vi "get current vi lib.vi"(8 "Stored Path":path) -> (0 "Current VI Lib Path":path)   [LabVIEW 2014, in "PL Framework Configuration Tool.lvlib"]
uses:
  PL Framework Configuration Tool.lvlib
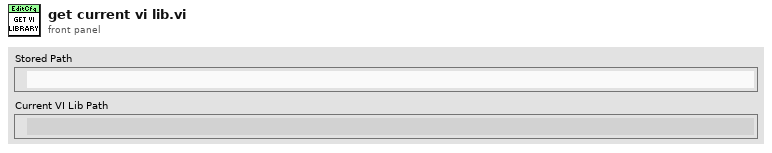
[diagram p1: front panel]
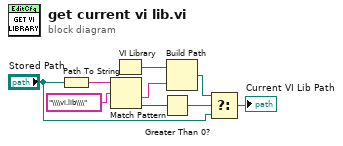
[diagram p0: block diagram]
diagram:
  n1 = Path To String(path="Stored Path") -> (string=w6:string)
  n2 = Match Pattern(string=w6, regular expression="\\\\vi.lib\\\\") -> (after substring=w7:string, offset past match=w5:i32)  [unwired: 1 in, 2 out]
  n3 = VI Library() -> (path=w8:path)
  n4 = Greater Than 0?(x=w5) -> (x > 0?=w4:bool)
  n5 = Build Path(base path=w8, name or relative path=w7) -> (appended path=w3:path)
  n6 = Select(t=w3, s=w4, f="Stored Path") -> (s? t:f=→"Current VI Lib Path":path)
